vi "Material-Line3-TestMain.vi"(8 "error in (no error)":errorcluster, 11 "Material-RunTest in":refnum<class "Material-RunTest.lvclass">) -> (0 "error out":errorcluster, 3 "Material-RunTest out":refnum<class "Material-RunTest.lvclass">)   [LabVIEW 2013, in "Material-RunTest.lvclass"]
uses:
  Material-RunTest.lvclass
  Material-RunTest.lvclass/Material-RunTest.ctl
  Motion Control/Motion-ControlAll.lvclass
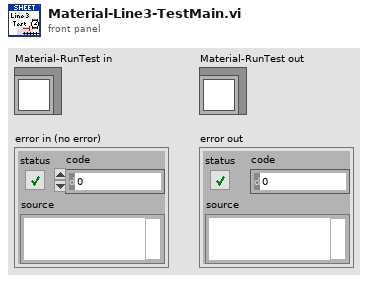
[diagram p1: front panel]
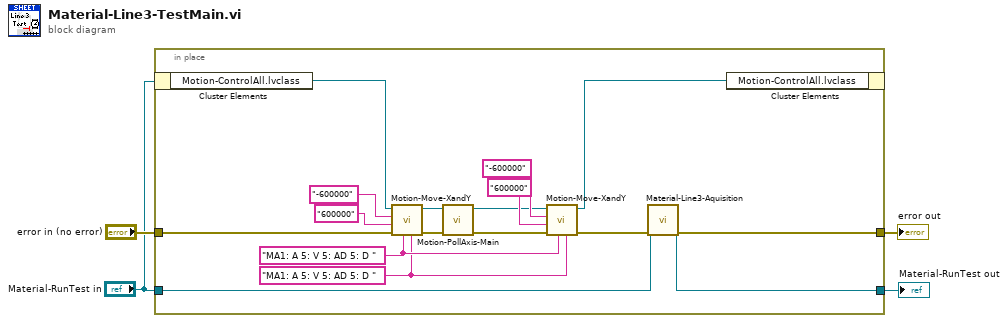
[diagram p0: block diagram]
diagram:
  n1 = in-place {
    in-place-border: "error in (no error)" -> [w21]
    in-place-border: [w6] -> w4
    in-place-border: "Material-RunTest in" -> [w7]
    in-place-border: [w5] -> w1
    w9 = "MA1: A 5: V 5: AD 5: D " ("concatenated string")
    w10 = "MA1: A 5: V 5: AD 5: D " ("concatenated string")
    n2 = in-place-cluster #1("Material-RunTest in") -> ("Motion-ControlAll.lvclass"=w20:refnum<class "Motion-ControlAll.lvclass">)
    n3 = call "Motion-Move-XandY.vi"("Y Drive Acc/Speed/Velocity"=w9, "X Drive Acc/Speed/Velocity"=w10, "error in (no error)"=w21, "X Coordinates"="600000", "Y Coordinates"="-600000", "Motion-ControlAll in"=w20) -> ("error out"=w18:errorcluster, "Motion-ControlAll out"=w19:refnum<class "Motion-ControlAll.lvclass">)  [unwired: 4 in]
    n4 = call "Motion-PollAxis-Main.vi"("error in (no error)"=w18, "Motion-ControlAll in"=w19) -> ("error out"=w13:errorcluster, "Motion-ControlAll out"=w12:refnum<class "Motion-ControlAll.lvclass">)  [unwired: 8 in]
    n5 = call "Motion-Move-XandY.vi"("Y Drive Acc/Speed/Velocity"=w9, "X Drive Acc/Speed/Velocity"=w10, "error in (no error)"=w13, "X Coordinates"="600000", "Y Coordinates"="-600000", "Motion-ControlAll in"=w12) -> ("error out"=w8:errorcluster, "Motion-ControlAll out"=w11:refnum<class "Motion-ControlAll.lvclass">)  [unwired: 4 in]
    n6 = call "Material-Line3-Aquisition.vi"("error in (no error)"=w8, "Material-RunTest in"=w7) -> ("error out"=w6:errorcluster, "Material-RunTest out"=w5:refnum<class "Material-RunTest.lvclass">)  [unwired: 8 in]
    n7 = in-place-cluster #1("Motion-ControlAll.lvclass"=w11) -> ()  [unwired: 1 out]
  }
  "Material-RunTest out" <- w1
  "error out" <- w4
